vi "VFD.vi"() -> (0 "GS1 Communication Error Out":errorcluster)   [LabVIEW 2017]
uses:
  timing_clust.ctl
  nitl_modes.ctl
  wakeup.ctl
  MB Serial Master Query Write Single Register (poly).vi
  XDataNode.xnode
  XDNodeRunTimeDep.lvlib
  MB Serial Master Query Read Holding Registers (poly).vi
panel:
  in  "VFD Stop":bool
  in  "GS1 Communication Error In":errorcluster
  out "Iteration Duration":i64
  out "Finished Late? [i-1]":bool
  out "TCHX Initializaton Error":errorcluster
  out "TCHX Initialization Loop Time (ms)":u32
  out "CTAH Initializaton Error":errorcluster
  out "CTAH Initialization Loop Time (ms)":u32
  out "Pump Initializaton Error":errorcluster
  out "Pump Initialization Loop Time (ms)":u32
  in  "Starting Address":u16
  out "Holding Registers":u16[](array[numeric])
  out "error out":errorcluster
  out "VISA resource name out":refnum<visa-resource-name>
  out "400001":u16
  out "error out":errorcluster
  # "Troubleshooting Modbus communication using third-party VIs and native I/O Server"
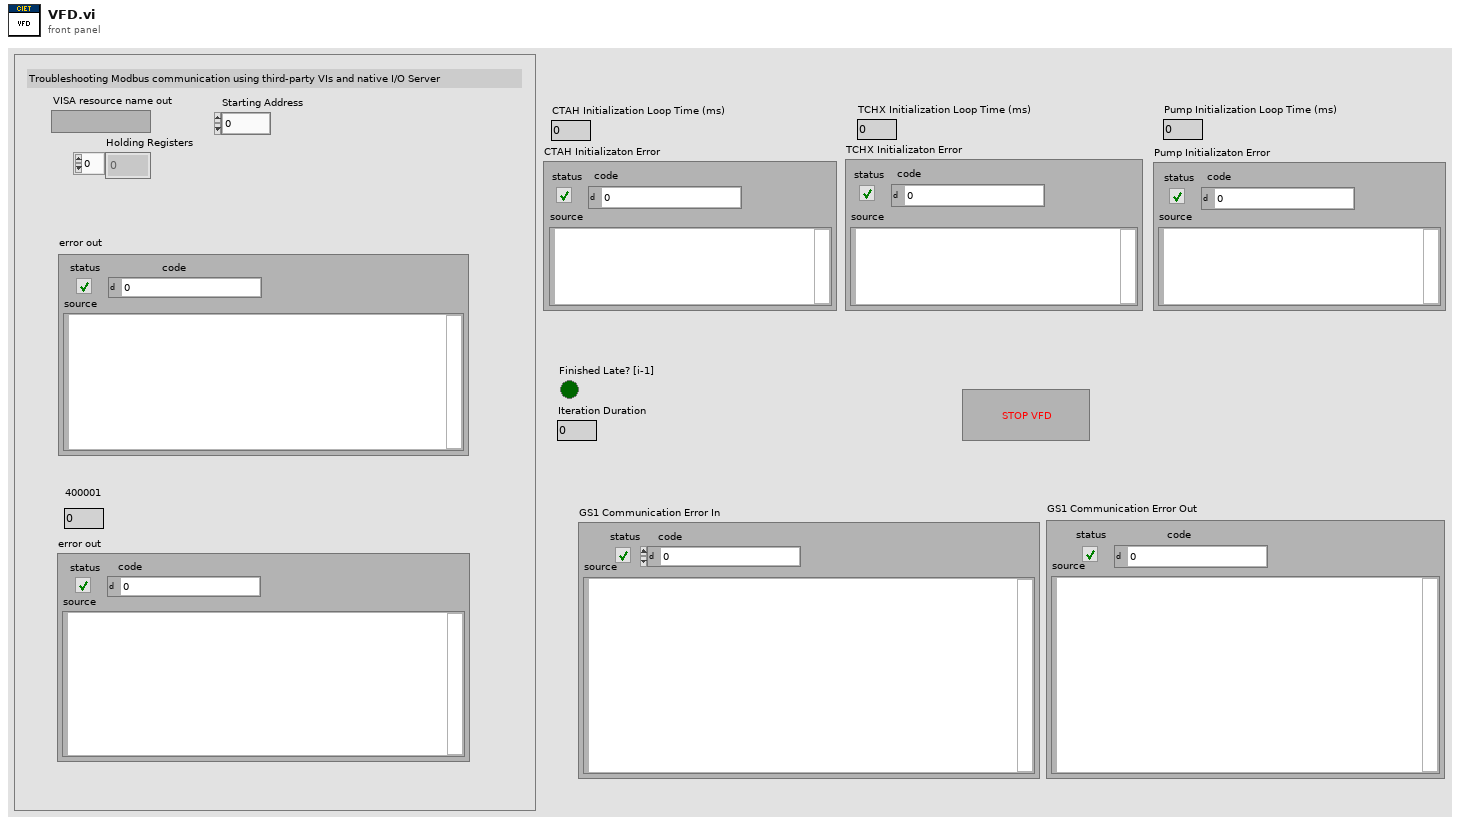
[diagram p1: front panel]
types:
  T1 = cluster{"Mode":enum16{"RTU", "ASCII"}, "Slave Address":u8}
  T2 = typedef "XDNodeRunTimeDep.lvlib/timing_clust.ctl" = cluster{"Expected End [f-1]":u64, "Actual End [f-1]":u64, "Finished Late? [f-1]":bool, "Expected End [i-1]":u64, "Actual End [i-1]":u64, "Finished Late? [i-1]":bool, "Expected Start [i]":u64, "Actual Start [i]":u64, "Expected Start [f]":u64, "Actual Start [f]":u64, "Source Name":string, "Structure Name":string, "Period":i64, "Deadline":i64, "Offset":i64, "Start":i64, "Priority":i32, "Timeout":i32, "Mode":T3, "Wakeup Reason":T4, "Error":errorcluster, "Source Type":string, "Secondary Source Type":string, "Global End Time":u64, "Global Start Time":u64, "Frame Duration":u64, "Iteration Duration":u64, "Assigned CPU":i32, "I/O Scan Engine Mode":u32}
  T3 = typedef "XDNodeRunTimeDep.lvlib/nitl_modes.ctl" = enum32{"No Change", "Process missed periods, maintain original phase", "Discard missed periods, maintain original phase", "Process missed periods, ignore original phase", "Discard missed periods, ignore original phase"}
  T4 = typedef "XDNodeRunTimeDep.lvlib/wakeup.ctl" = enum32{"Normal", "Aborted", "Asynchronous wakeup", "Timing source error", "Timed loop error", "Timeout"}
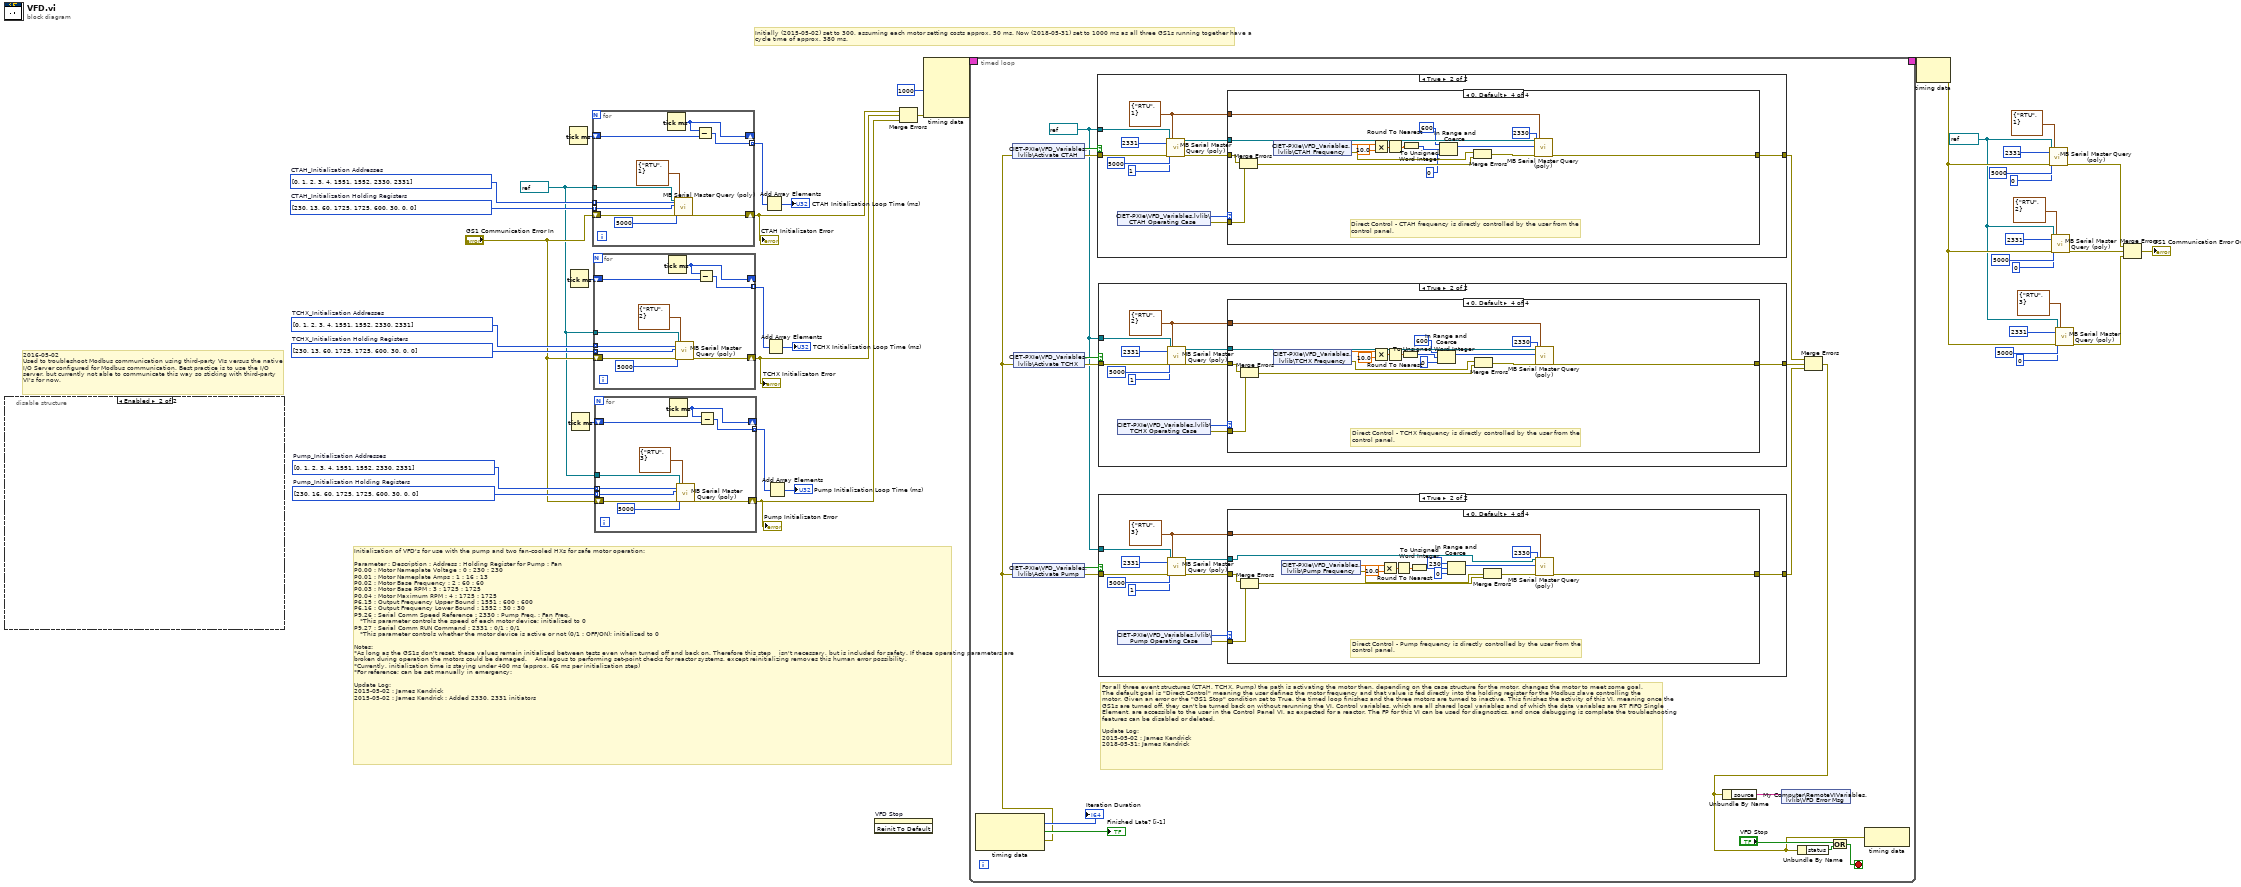
[diagram p0: block diagram]
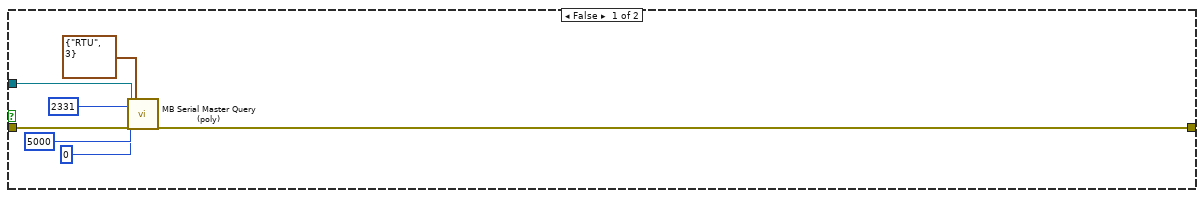
[diagram p2: hidden frame]
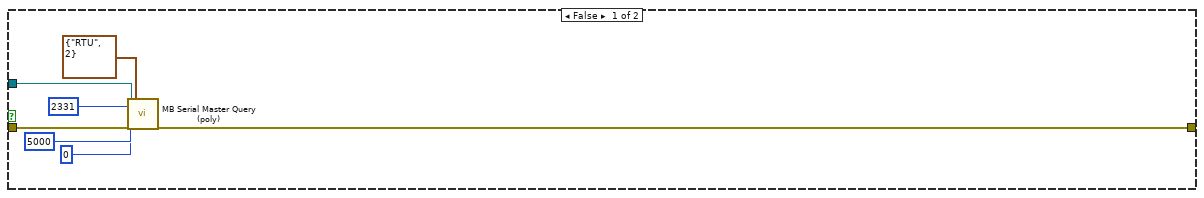
[diagram p6: hidden frame]
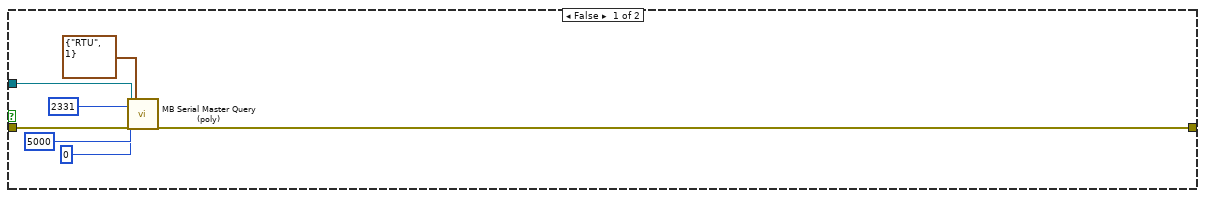
[diagram p10: hidden frame]
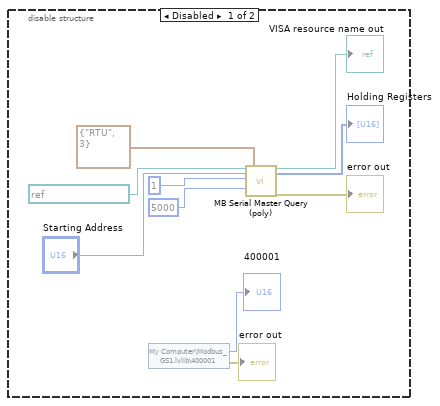
[diagram p14: hidden frame]
diagram:
  w4 = refnum<visa-resource-name> "VFD" ("VISA resource name")
  w5 = refnum<visa-resource-name> "VFD" ("VISA resource name")
  w28 = u16[] [230, 13, 60, 1725, 1725, 600, 30, 0, 0]  # TCHX_Initialization Holding Registers
  w29 = u16[] [0, 1, 2, 3, 4, 1551, 1552, 2330, 2331]  # TCHX_Initialization Addresses
  w33 = u16[] [230, 13, 60, 1725, 1725, 600, 30, 0, 0]  # CTAH_Initialization Holding Registers
  w34 = u16[] [0, 1, 2, 3, 4, 1551, 1552, 2330, 2331]  # CTAH_Initialization Addresses
  w41 = u16[] [230, 16, 60, 1725, 1725, 600, 30, 0, 0]  # Pump_Initialization Holding Registers
  w42 = u16[] [0, 1, 2, 3, 4, 1551, 1552, 2330, 2331]  # Pump_Initialization Addresses
  # "Initially (2015-05-02) set to 300, assuming each motor setting costs approx. 50 ms. Now (2018-05-31) set to 1000 ms as all three GS1s running together have a \ncycle time of approx. 380 ms."
  # "2016-05-02\nUsed to troubleshoot Modbus communication using third-party VIs versus the native\nI/O Server configured for Modbus communication. Best practice is to use the I/O \nserver, but currently not able to communicate this way so sticking with third-party \nVI's for now."
  # "Initialization of VFD's for use with the pump and two fan-cooled HXs for safe motor operation:\n\nParameter : Description : Address : Holding Register for Pump : Fan\nP0.00 : Motor Nameplate Voltage : 0 : 230 : 230\nP0.01 : Motor Nameplate Amps : 1 : 16 : 13\nP0.02 : Motor Base Frequency : 2 : 60 : 60\nP0.03 : Motor Base RPM : 3 : 1725 : 1725\nP0.04 : Motor Maximum RPM : 4 : 1725 : 1725\nP6.15 : Output Frequency Upper Bound : 1551 : 600 : 600\nP6.16 : Output Frequency Lower Bound : 1552 : 30 : 30\nP9.26 : Serial Comm Speed Reference : 2330 : Pump Freq. : Fan Freq. \n   *This parameter controls the speed of each motor device; initialized to 0\nP9.27 : Serial Comm RUN Command : 2331 : 0/1 : 0/1\n   *This parameter controls whether the motor device is active or not (0/1 : OFF/ON); initialized to 0\n\nNotes:\n*As long as the GS1s don't reset, these values remain initialized between tests even when turned off and back on. Therefore this step    isn't necessary, but is included for safety. If these operating parameters are broken during operation the motors could be damaged.    Analagous to performing set-point checks for reactor systems, except reinitializing removes this human error possibility.\n*Currently, initialization time is staying under 400 ms (approx. 66 ms per initialization step)\n*For reference; can be set manually in emergency:\n\nUpdate Log:\n2015-05-02 : James Kendrick \n2015-05-02 : James Kendrick : Added 2330, 2331 initiators"
  n1 = disable-structure shown="Enabled" {
    frame Disabled {
      n2 = shared-variable "My Computer\\Modbus_GS1.lvlib\\400001"() -> (→"400001":u16, error out=→"error out":errorcluster)  [unwired: 1 in]
      n3 = call-poly "MB Serial Master Query (poly).vi"("VISA resource name"=refnum<visa-resource-name> "GS1_AC_Drive", "Starting Address"="Starting Address", "Quantity"=u16 1, "Timeout"=u32 5000, "Serial Parameters"=T1 {"Mode"=enum."RTU", "Slave Address"=3}) -> ("VISA resource name out"=→"VISA resource name out":refnum<visa-resource-name>, "Holding Registers"=→"Holding Registers":u16[], "error out"=→"error out":errorcluster)  [unwired: 11 in, 1 out]
    }
    frame Enabled {
    }
  }
  n4 = Tick Count (ms)() -> (millisecond timer value=w32:u32)
  n5 = Tick Count (ms)() -> (millisecond timer value=w27:u32)
  n6 = Tick Count (ms)() -> (millisecond timer value=w40:u32)
  n7 = for {
    shift-right: [w60] -> w13
    shift-left: "GS1 Communication Error In" -> [w61]
    tunnel: w34 -> [w59] mode=indexing
    tunnel: w33 -> [w58] mode=indexing
    shift-right: [w55] -> _
    shift-left: w32 -> [w57]
    tunnel: [w56] -> w31 mode=indexing
    tunnel: w5 -> [w54]
    n8 = Tick Count (ms)() -> (millisecond timer value=w55:u32)
    n9 = call-poly "MB Serial Master Query (poly).vi"("VISA resource name"=w54, "Address"=w59, "Holding Register"=w58, "Timeout"=u32 5000, "error in"=w61, "Serial Parameters"=T1 {"Mode"=enum."RTU", "Slave Address"=1}) -> ("error out"=w60:errorcluster)  [unwired: 11 in, 2 out]
    n10 = Subtract(x=w55, y=w57) -> (x-y=w56:u32)
  }
  "CTAH Initializaton Error" <- w13
  n11 = for {
    shift-right: [w70] -> w7
    shift-left: "GS1 Communication Error In" -> [w71]
    tunnel: w29 -> [w69] mode=indexing
    tunnel: w28 -> [w68] mode=indexing
    shift-right: [w65] -> _
    shift-left: w27 -> [w67]
    tunnel: [w66] -> w26 mode=indexing
    tunnel: w5 -> [w64]
    n12 = Tick Count (ms)() -> (millisecond timer value=w65:u32)
    n13 = call-poly "MB Serial Master Query (poly).vi"("VISA resource name"=w64, "Address"=w69, "Holding Register"=w68, "Timeout"=u32 5000, "error in"=w71, "Serial Parameters"=T1 {"Mode"=enum."RTU", "Slave Address"=2}) -> ("error out"=w70:errorcluster)  [unwired: 11 in, 2 out]
    n14 = Subtract(x=w65, y=w67) -> (x-y=w66:u32)
  }
  "TCHX Initializaton Error" <- w7
  n15 = for {
    shift-right: [w80] -> w6
    shift-left: "GS1 Communication Error In" -> [w81]
    tunnel: w42 -> [w79] mode=indexing
    tunnel: w41 -> [w78] mode=indexing
    shift-right: [w75] -> _
    shift-left: w40 -> [w77]
    tunnel: [w76] -> w39 mode=indexing
    tunnel: w5 -> [w74]
    n16 = Tick Count (ms)() -> (millisecond timer value=w75:u32)
    n17 = call-poly "MB Serial Master Query (poly).vi"("VISA resource name"=w74, "Address"=w79, "Holding Register"=w78, "Timeout"=u32 5000, "error in"=w81, "Serial Parameters"=T1 {"Mode"=enum."RTU", "Slave Address"=3}) -> ("error out"=w80:errorcluster)  [unwired: 11 in, 2 out]
    n18 = Subtract(x=w75, y=w77) -> (x-y=w76:u32)
  }
  "Pump Initializaton Error" <- w6
  n19 = Add Array Elements(numeric array=w31) -> (sum=→"CTAH Initialization Loop Time (ms)":u32)
  n20 = Add Array Elements(numeric array=w26) -> (sum=→"TCHX Initialization Loop Time (ms)":u32)
  n21 = Add Array Elements(numeric array=w39) -> (sum=→"Pump Initialization Loop Time (ms)":u32)
  n22 = invoke on="VFD Stop" class="Bool (strict)" method="Reinit To Default"() -> ()  [unwired: 3 in, 3 out]
  n23 = Merge Errors(w13, w7, w6) -> (w15:errorcluster)
  n24 = node-c288(i64 1000 ("Pump Control Period (ms)"), w15) -> (w37:T2)  [unwired: 3 in]
  n25 = timed-loop {
    timing: w37 -> [_]
    timing-out: [_] -> w36
    stop <- w96 stop-if-true
    w86 = refnum<visa-resource-name> "VFD" ("VISA resource name")
    # "For all three event structures (CTAH, TCHX, Pump) the path is activating the motor then, depending on the case structure for the motor, changes the motor to meet some goal. \nThe default goal is \"Direct Control\" meaning the user defines the motor frequency and that value is fed directly into the holding register for the Modbus slave controlling the \nmotor. Given an error or the \"GS1 Stop\" condition set to True, the timed loop finishes and the three motors are turned to inactive. This finishes the activity of this VI, meaning once the\nGS1s are turned off, they can't be turned back on without rerunning the VI. Control variables, which are all shared local variables and of which the data variables are RT FIFO Single\nElement, are accessible to the user in the Control Panel VI, as expected for a reactor. The FP for this VI can be used for diagnostics, and once debugging is complete the troubleshooting\nfeatures can be disabled or deleted.  \n\nUpdate Log:\n2015-05-02 : James Kendrick\n2018-05-31: James Kendrick"
    n26 = node-c288() -> (→"Iteration Duration":i64, →"Finished Late? [i-1]":bool, w90:errorcluster)  [unwired: 1 in]
    n27 = shared-variable "CIET-PXIe\\VFD_Variables.lvlib\\Activate CTAH"(error in=w90) -> (w100:bool, error out=w99:errorcluster)
    n28 = shared-variable "CIET-PXIe\\VFD_Variables.lvlib\\Activate Pump"(error in=w90) -> (w93:bool, error out=w92:errorcluster)
    n29 = shared-variable "CIET-PXIe\\VFD_Variables.lvlib\\Activate TCHX"(error in=w90) -> (w95:bool, error out=w94:errorcluster)
    n30 = case shown="True" w100 {
      tunnel: w99 -> [w174 w184]
      tunnel: [w173 w180] -> w89
      tunnel: w86 -> [w172 w179]
      frame False {
        n31 = call-poly "MB Serial Master Query (poly).vi"("VISA resource name"=w172, "Address"=u16 2331, "Holding Register"=u16 0, "Timeout"=u32 5000, "error in"=w174, "Serial Parameters"=T1 {"Mode"=enum."RTU", "Slave Address"=1}) -> ("error out"=w173:errorcluster)  [unwired: 11 in, 2 out]
      }
      frame True {
        w178 = T1 {"Mode"=enum."RTU", "Slave Address"=1} ("Serial Parameters")
        n32 = shared-variable "CIET-PXIe\\VFD_Variables.lvlib\\CTAH Operating Case"() -> (w182:i32, error out=w181:errorcluster)  [unwired: 1 in]
        n33 = call-poly "MB Serial Master Query (poly).vi"("VISA resource name"=w179, "Address"=u16 2331, "Holding Register"=u16 1, "Timeout"=u32 5000, "error in"=w184, "Serial Parameters"=w178) -> ("VISA resource name out"=w183:refnum<visa-resource-name>, "error out"=w185:errorcluster)  [unwired: 11 in, 1 out]
        n34 = case shown="0, Default" w182 {
          tunnel: w185 -> [_ _ _ w204]
          tunnel: w183 -> [_ _ _ w205]
          tunnel: w181 -> [_ _ _ w203]
          tunnel: [_ _ _ w199] -> w180
          tunnel: w178 -> [_ _ _ w198]
          frame 1 {
            # "CTAH Outlet Temp: Feedback - CTAH frequency is determined by a\ncontrol function to hold the outlet temperature of the CTAH \nconstant."
          }
          frame 2 {
            # "Load Following - CTAH frequency is controlled to make the CTAH heat removal power\nto equal a user specified value through satisfying the equation: m_dot*c_P*(T_in - T_out)"
          }
          frame 3 {
            # "Dynamic Forcing - CTAH frequency is defined by a waveform function to drive the \nCTAH frequency and thus mass flow rate in a dynamic pattern, such as a square wave,\nsine wave, or other function as defined by the user.\n\nUser inputs to include:\nCTAH frequency set point (used as signal offset)\nSignal amplitude\nSignal frequency\nSignal type: sine, square, others?"
          }
          frame 0, Default {
            # "Direct Control - CTAH frequency is directly controlled by the user from the\ncontrol panel."
            n35 = Merge Errors(w204, w203) -> (w200:errorcluster)
            n36 = shared-variable "CIET-PXIe\\VFD_Variables.lvlib\\CTAH Frequency"() -> (w195:sgl, error out=w196:errorcluster)  [unwired: 1 in]
            n37 = Multiply(x=w195, y=sgl 10.0) -> (x*y=w197:sgl)
            n38 = Round To Nearest(number=w197) -> (nearest integer value=w194:sgl)
            n39 = To Unsigned Word Integer(number=w194) -> (unsigned 16bit integer=w192:u16)
            n40 = In Range and Coerce(upper limit=u16 600, x=w192, lower limit=u16 0) -> (coerced(x)=w191:u16)  [unwired: 1 out]
            n41 = Merge Errors(w196, w200) -> (w201:errorcluster)
            n42 = call-poly "MB Serial Master Query (poly).vi"("VISA resource name"=w205, "Address"=u16 2330, "Holding Register"=w191, "error in"=w201, "Serial Parameters"=w198) -> ("error out"=w199:errorcluster)  [unwired: 12 in, 2 out]
          }
        }
      }
    }
    n43 = case shown="True" w95 {
      tunnel: w94 -> [w139 w149]
      tunnel: [w138 w145] -> w88
      tunnel: w86 -> [w137 w144]
      frame False {
        n44 = call-poly "MB Serial Master Query (poly).vi"("VISA resource name"=w137, "Address"=u16 2331, "Holding Register"=u16 0, "Timeout"=u32 5000, "error in"=w139, "Serial Parameters"=T1 {"Mode"=enum."RTU", "Slave Address"=2}) -> ("error out"=w138:errorcluster)  [unwired: 11 in, 2 out]
      }
      frame True {
        w143 = T1 {"Mode"=enum."RTU", "Slave Address"=2} ("Serial Parameters")
        n45 = shared-variable "CIET-PXIe\\VFD_Variables.lvlib\\TCHX Operating Case"() -> (w147:i32, error out=w146:errorcluster)  [unwired: 1 in]
        n46 = call-poly "MB Serial Master Query (poly).vi"("VISA resource name"=w144, "Address"=u16 2331, "Holding Register"=u16 1, "Timeout"=u32 5000, "error in"=w149, "Serial Parameters"=w143) -> ("VISA resource name out"=w148:refnum<visa-resource-name>, "error out"=w150:errorcluster)  [unwired: 11 in, 1 out]
        n47 = case shown="0, Default" w147 {
          tunnel: w150 -> [_ _ _ w169]
          tunnel: w148 -> [_ _ _ w170]
          tunnel: w146 -> [_ _ _ w168]
          tunnel: [_ _ _ w164] -> w145
          tunnel: w143 -> [_ _ _ w163]
          frame 1 {
            # "TCHX Outlet Temp: Feedback - TCHX frequency is determined by a\ncontrol function to hold the outlet temperature of the TCHX \nconstant."
          }
          frame 2 {
            # "Freezing Event - TCHX frequency is adjust to simulate a freezing transient or freeze\nevent within the TCHX, compromising the heat transfer path from the core to\nenvironment during a transient without use of the pump/CTAH."
          }
          frame 3 {
            # "Dynamic Forcing - TCHX frequency is defined by a waveform function to drive the \nTCHX frequency and thus mass flow rate in a dynamic pattern, such as a square wave,\nsine wave, or other function as defined by the user.\n\nUser inputs to include:\nTCHX frequency set point (used as signal offset)\nSignal amplitude\nSignal frequency\nSignal type: sine, square, others?"
          }
          frame 0, Default {
            # "Direct Control - TCHX frequency is directly controlled by the user from the\ncontrol panel."
            n48 = Merge Errors(w169, w168) -> (w165:errorcluster)
            n49 = shared-variable "CIET-PXIe\\VFD_Variables.lvlib\\TCHX Frequency"() -> (w162:sgl, error out=w158:errorcluster)  [unwired: 1 in]
            n50 = Multiply(x=w162, y=sgl 10.0) -> (x*y=w161:sgl)
            n51 = Round To Nearest(number=w161) -> (nearest integer value=w160:sgl)
            n52 = To Unsigned Word Integer(number=w160) -> (unsigned 16bit integer=w156:u16)
            n53 = In Range and Coerce(upper limit=u16 600, x=w156, lower limit=u16 0) -> (coerced(x)=w157:u16)  [unwired: 1 out]
            n54 = Merge Errors(w158, w165) -> (w166:errorcluster)
            n55 = call-poly "MB Serial Master Query (poly).vi"("VISA resource name"=w170, "Address"=u16 2330, "Holding Register"=w157, "error in"=w166, "Serial Parameters"=w163) -> ("error out"=w164:errorcluster)  [unwired: 12 in, 2 out]
          }
        }
      }
    }
    n56 = case shown="True" w93 {
      tunnel: w92 -> [w104 w114]
      tunnel: [w103 w110] -> w87
      tunnel: w86 -> [w102 w109]
      frame False {
        n57 = call-poly "MB Serial Master Query (poly).vi"("VISA resource name"=w102, "Address"=u16 2331, "Holding Register"=u16 0, "Timeout"=u32 5000, "error in"=w104, "Serial Parameters"=T1 {"Mode"=enum."RTU", "Slave Address"=3}) -> ("error out"=w103:errorcluster)  [unwired: 11 in, 2 out]
      }
      frame True {
        w108 = T1 {"Mode"=enum."RTU", "Slave Address"=3} ("Serial Parameters")
        n58 = shared-variable "CIET-PXIe\\VFD_Variables.lvlib\\Pump Operating Case"() -> (w112:i32, error out=w111:errorcluster)  [unwired: 1 in]
        n59 = call-poly "MB Serial Master Query (poly).vi"("VISA resource name"=w109, "Address"=u16 2331, "Holding Register"=u16 1, "Timeout"=u32 5000, "error in"=w114, "Serial Parameters"=w108) -> ("VISA resource name out"=w113:refnum<visa-resource-name>, "error out"=w115:errorcluster)  [unwired: 11 in, 1 out]
        n60 = case shown="0, Default" w112 {
          tunnel: w115 -> [_ _ _ w135]
          tunnel: w113 -> [_ _ _ w125]
          tunnel: w111 -> [_ _ _ w134]
          tunnel: [_ _ _ w130] -> w110
          tunnel: w108 -> [_ _ _ w124]
          frame 1 {
            # "Mass Flow Rate: Feedback - Pump frequency is controlled through \na closed feedback to match a specified mass flow rate defined by \nthe user on the control panel."
          }
          frame 2 {
            # "Mass Flow Rate: Ramp - Pump frequency is controlled through a control function that\ncontrols the rate of change of the mass flow rate that the user specifies on the control\npanel to match a user desired final mass flow rate."
          }
          frame 3 {
            # "Dynamic Forcing - Pump frequency is defined by a waveform function to drive the \npump frequency and thus mass flow rate in a dynamic pattern, such as a square wave,\nsine wave, or other function as defined by the user.\n\nUser inputs to include:\nPump frequency set point (used as signal offset)\nSignal amplitude\nSignal frequency\nSignal type: sine, square, others?"
          }
          frame 0, Default {
            # "Direct Control - Pump frequency is directly controlled by the user from the\ncontrol panel."
            n61 = Merge Errors(w135, w134) -> (w131:errorcluster)
            n62 = shared-variable "CIET-PXIe\\VFD_Variables.lvlib\\Pump Frequency"() -> (w122:sgl, error out=w126:errorcluster)  [unwired: 1 in]
            n63 = Multiply(x=w122, y=sgl 10.0) -> (x*y=w123:sgl)
            n64 = Round To Nearest(number=w123) -> (nearest integer value=w120:sgl)
            n65 = To Unsigned Word Integer(number=w120) -> (unsigned 16bit integer=w119:u16)
            n66 = In Range and Coerce(upper limit=u16 230, x=w119, lower limit=u16 0) -> (coerced(x)=w127:u16)  [unwired: 1 out]
            n67 = Merge Errors(w126, w131) -> (w132:errorcluster)
            n68 = call-poly "MB Serial Master Query (poly).vi"("VISA resource name"=w125, "Address"=u16 2330, "Holding Register"=w127, "error in"=w132, "Serial Parameters"=w124) -> ("error out"=w130:errorcluster)  [unwired: 12 in, 2 out]
          }
        }
      }
    }
    n69 = Merge Errors(w89, w88, w87) -> (w84:errorcluster)
    n70 = Unbundle By Name(w84) -> ("source"=w83:string)
    n71 = shared-variable "My Computer\\RemoteVIVariables.lvlib\\VFD Error Msg"(w83) -> ()  [unwired: 1 in, 1 out]
    n72 = Unbundle By Name(w84) -> ("status"=w91:bool)
    n73 = Or(x="VFD Stop", y=w91) -> (x .or. y?=w96:bool)
    n74 = node-c288(w84) -> ()  [unwired: 1 out]
  }
  n75 = node-c288(w36) -> (w8:errorcluster)
  n76 = call-poly "MB Serial Master Query (poly).vi"("VISA resource name"=w4, "Address"=u16 2331, "Holding Register"=u16 0, "Timeout"=u32 5000, "error in"=w8, "Serial Parameters"=T1 {"Mode"=enum."RTU", "Slave Address"=1}) -> ("error out"=w10:errorcluster)  [unwired: 11 in, 2 out]
  n77 = call-poly "MB Serial Master Query (poly).vi"("VISA resource name"=w4, "Address"=u16 2331, "Holding Register"=u16 0, "Timeout"=u32 5000, "error in"=w8, "Serial Parameters"=T1 {"Mode"=enum."RTU", "Slave Address"=2}) -> ("error out"=w11:errorcluster)  [unwired: 11 in, 2 out]
  n78 = call-poly "MB Serial Master Query (poly).vi"("VISA resource name"=w4, "Address"=u16 2331, "Holding Register"=u16 0, "Timeout"=u32 5000, "error in"=w8, "Serial Parameters"=T1 {"Mode"=enum."RTU", "Slave Address"=3}) -> ("error out"=w9:errorcluster)  [unwired: 11 in, 2 out]
  n79 = Merge Errors(w10, w11, w9) -> (→"GS1 Communication Error Out":errorcluster)
